vi "AutoCAD cmds.vi"(6 "AutoCAD cmd":T4, 8 "error in (no error)":errorcluster, 11 "UserInputs":T3) -> (0 "error out":errorcluster, 2 "IsQuiescent":bool)   [LabVIEW 2015, in "AguaClara Library.lvlib"]
uses:
  AguaClara Library.lvlib
  AutoCAD cmds.ctl
  user project design.ctl
  Variable cluster.ctl
  Design Request.ctl
panel:
  in  "Mathcad Output":T1
  out "DesignRequest out":T2
  in  "DesignRequest":T2
  out "new doc error":errorcluster
  out "Iterations":i32
  out "Visible":bool
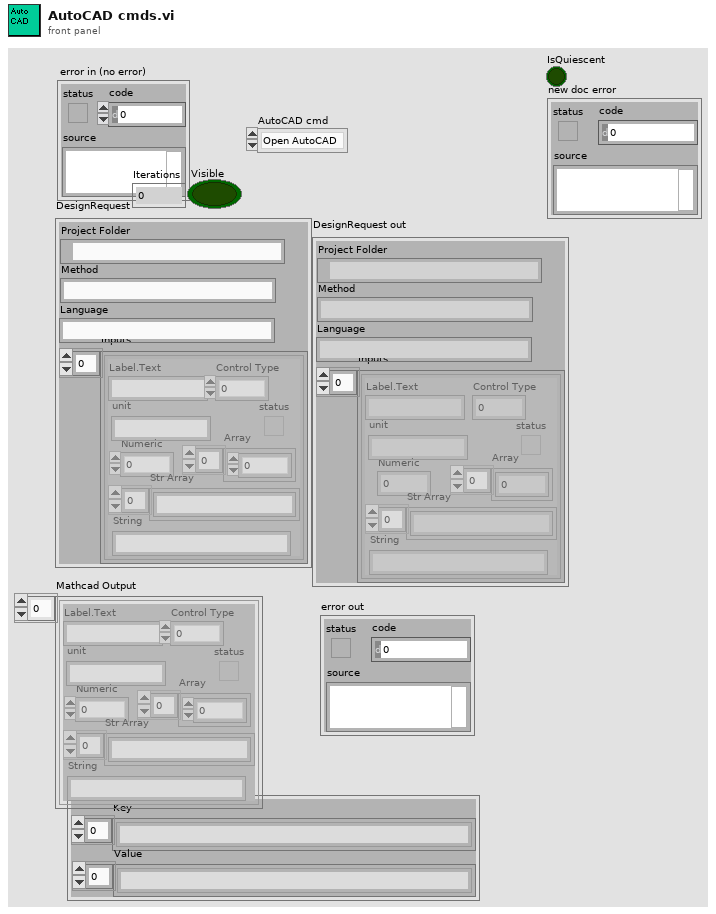
[diagram p1: front panel]
types:
  T1 = typedef "Variable cluster.ctl" = cluster{"Label.Text":string, "Control Type":u32, "Numeric":dbl, "Array":dbl[], "status":bool, "Str Array":string[], "String":string, "unit":string}[]
  T2 = typedef "Design Request.ctl" = cluster{"Project Folder":path, "Method":string, "Inputs":T1, "Language":string}
  T3 = typedef "user project design.ctl" = cluster{"Key":string[], "Value":string[]}
  T4 = typedef "AguaClara Library.lvlib/AutoCAD cmds.ctl" = enum16{"Open AutoCAD", "New Document", "Send Command", "Send Command Array", "Close Doc", "Quit"}
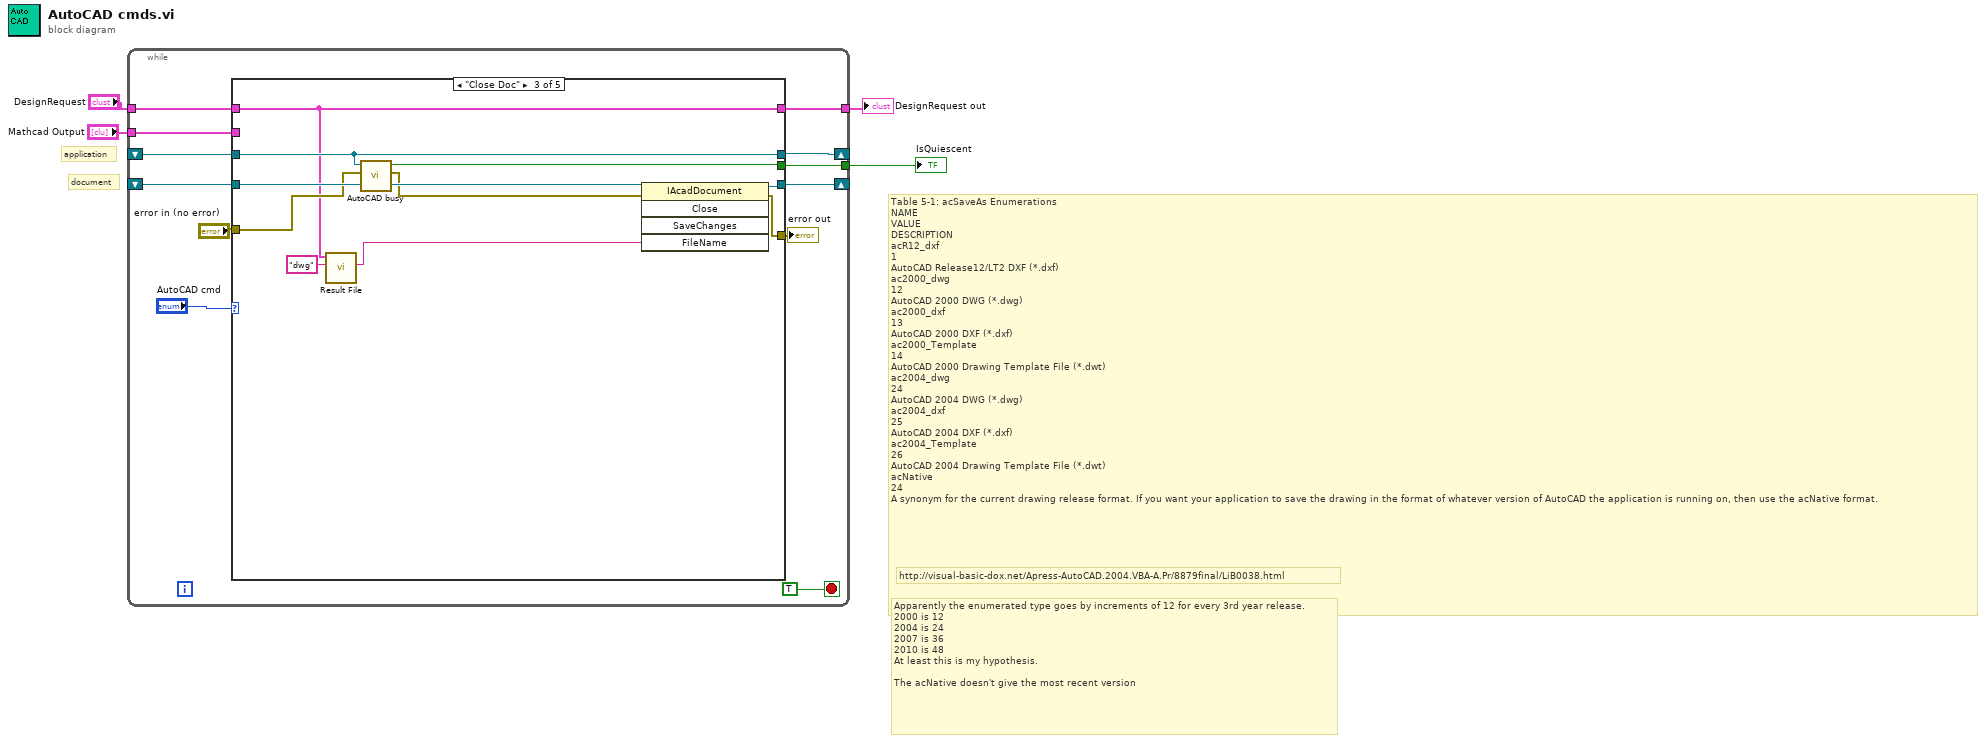
[diagram p0: block diagram]
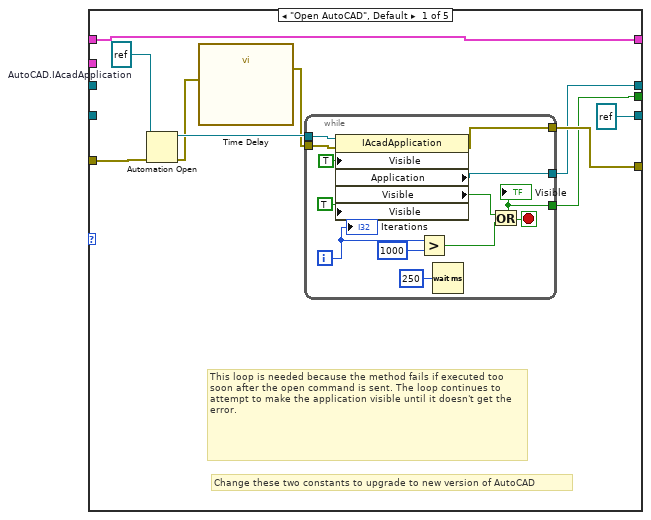
[diagram p2: hidden frame]
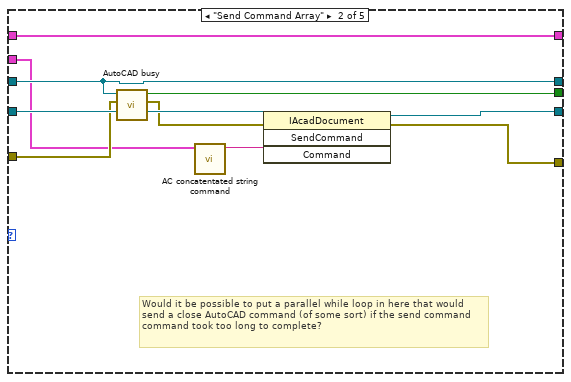
[diagram p3: hidden frame]
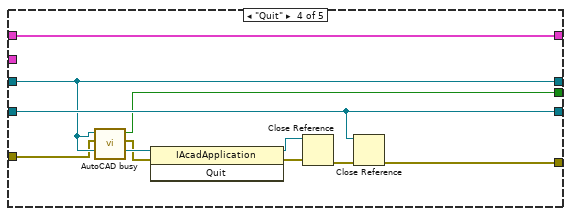
[diagram p4: hidden frame]
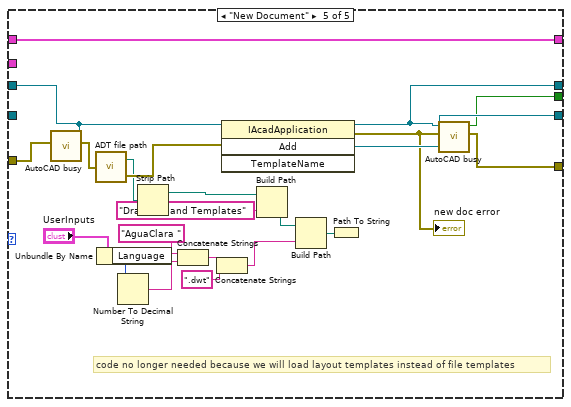
[diagram p5: hidden frame]
diagram:
  # "Apparently the enumerated type goes by increments of 12 for every 3rd year release.\n2000 is 12\n2004 is 24\n2007 is 36\n2010 is 48\nAt least this is my hypothesis. \n\nThe acNative doesn't give the most recent version"
  # "http://visual-basic-dox.net/Apress-AutoCAD.2004.VBA-A.Pr/8879final/LiB0038.html"
  # "Table 5-1: acSaveAs Enumerations\nNAME\nVALUE\nDESCRIPTION\nacR12_dxf\n1\nAutoCAD Release12/LT2 DXF (*.dxf)\nac2000_dwg\n12\nAutoCAD 2000 DWG (*.dwg)\nac2000_dxf\n13\nAutoCAD 2000 DXF (*.dxf)\nac2000_Template\n14\nAutoCAD 2000 Drawing Template File (*.dwt)\nac2004_dwg\n24\nAutoCAD 2004 DWG (*.dwg)\nac2004_dxf\n25\nAutoCAD 2004 DXF (*.dxf)\nac2004_Template\n26\nAutoCAD 2004 Drawing Template File (*.dwt)\nacNative\n24\nA synonym for the current drawing release format. If you want your application to save the drawing in the format of whatever version of AutoCAD the application is running on, then use the acNative format."
  # "document"
  # "application"
  n1 = while {
    shift-right: [w15] -> _
    shift-left: _ -> [w10]
    shift-right: [w12] -> _
    shift-left: _ -> [w11]
    tunnel: [w6] -> w4
    tunnel: "DesignRequest" -> [w7]
    tunnel: [w8] -> w2
    tunnel: "Mathcad Output" -> [w5]
    stop <- TRUE stop-if-true
    n2 = case shown="\"Close Doc\"" "AutoCAD cmd" {
      tunnel: [w21 w41 w55 w62 w87] -> w15
      tunnel: "error in (no error)" -> [w24 w45 w54 w61 w83]
      tunnel: [w22 w43 w56 w63 w86] -> w13
      tunnel: [refnum<k7> refnum ("AutoCAD.IAcadDocument") w47 w57 w64 w90] -> w12
      tunnel: w11 -> [_ w48 w58 w64 _]
      tunnel: w10 -> [_ w41 w55 w62 w88]
      tunnel: [w17 w39 w51 w68 w89] -> w8
      tunnel: w7 -> [w17 w39 w51 w68 w89]
      tunnel: [w20 w44 w52 w59 w85] -> w6
      tunnel: w5 -> [_ w40 _ _ _]
      frame "Open AutoCAD", Default {
        w25 = refnum<k7> refnum  # AutoCAD.IAcadApplication
        # "This loop is needed because the method fails if executed too soon after the open command is sent. The loop continues to attempt to make the application visible until it doesn't get the error."
        # "Change these two constants to upgrade to new version of AutoCAD"
        n3 = Automation Open(error in (no error)=w24, Automation Refnum=w25) -> (Automation Refnum=w23:refnum<k7>, error out=w19:errorcluster)  [unwired: 2 in]
        n4 = call "Time Delay"("error in (no error)"=w19) -> ("error out"=w18:errorcluster)  [unwired: 10 in]
        n5 = while {
          tunnel: w23 -> [w38]
          tunnel: w18 -> [w37]
          tunnel: [w32] -> w22
          tunnel: [w31] -> w21
          tunnel: [w28] -> w20
          i -> [w35]
          stop <- w36 stop-if-true
          n6 = property class="IAcadApplication"(reference=w38, error in=w37, "Visible"=TRUE, "Visible"=TRUE) -> (error out=w32:errorcluster, "Application"=w31:refnum<k7>, "Visible"=w28:bool)  [unwired: 1 out]
          "Visible" <- w28
          n7 = Greater?(x=w35, y=1000) -> (0:w33:bool)
          n8 = Wait (ms)(milliseconds to wait=u32 250) -> ()  [unwired: 1 out]
          n9 = Or(x=w28, y=w33) -> (x .or. y?=w36:bool)
          "Iterations" <- w35
        }
      }
      frame "Send Command Array" {
        # "Would it be possible to put a parallel while loop in here that would send a close AutoCAD command (of some sort) if the send command command took too long to complete?"
        n10 = call "AutoCAD busy.vi"("error in (no error)"=w45, "Application"=w41) -> ("error out"=w42:errorcluster, "IsQuiescent"=w44:bool)  [unwired: 4 in]
        n11 = call "AC concatentated string command.vi"("MathCAD results"=w40) -> ("AC concatenated string"=w46:string)  [unwired: 10 in]
        n12 = invoke class="IAcadDocument" method="SendCommand"(reference=w48, error in=w42, "Command"=w46) -> (reference out=w47:refnum<k7>, error out=w43:errorcluster)  [unwired: 1 in, 2 out]
      }
      frame "Close Doc" {
        n13 = call "Result File.vi"("File Type"="dwg", "DesignRequest"=w51) -> ("File string"=w49:string)  [unwired: 8 in, 1 out]
        n14 = call "AutoCAD busy.vi"("error in (no error)"=w54, "Application"=w55) -> ("error out"=w53:errorcluster, "IsQuiescent"=w52:bool)  [unwired: 4 in]
        n15 = invoke class="IAcadDocument" method="Close"(reference=w58, error in=w53, "FileName"=w49) -> (reference out=w57:refnum<k7>, error out=w56:errorcluster)  [unwired: 2 in, 3 out]
      }
      frame "Quit" {
        n16 = call "AutoCAD busy.vi"("error in (no error)"=w61, "Application"=w62) -> ("error out"=w60:errorcluster, "IsQuiescent"=w59:bool)  [unwired: 4 in]
        n17 = invoke class="IAcadApplication" method="Quit"(reference=w62, error in=w60) -> (reference out=w67:refnum<k7>, error out=w66:errorcluster)  [unwired: 1 in, 1 out]
        n18 = Close Reference(reference=w67, error in (no error)=w66) -> (error out=w65:errorcluster)
        n19 = Close Reference(reference=w64, error in (no error)=w65) -> (error out=w63:errorcluster)
      }
      frame "New Document" {
        # "code no longer needed because we will load layout templates instead of file templates"
        n20 = call "AutoCAD busy.vi"("error in (no error)"=w83, "Application"=w88) -> ("error out"=w82:errorcluster)  [unwired: 4 in, 1 out]
        n21 = call "ADT file path.vi"("error in"=w82) -> ("error out"=w81:errorcluster, "dup path"=w74:path)
        n22 = Unbundle By Name("UserInputs") -> ("Language"=w80:enum16{"English", "Español", "French"})
        n23 = Number To Decimal String(number=w80) -> (decimal integer string=w78:string)  [unwired: 1 in]
        n24 = Strip Path(path=w74) -> (stripped path=w73:path)  [unwired: 1 out]
        n25 = Concatenate Strings("AguaClara " ("section"), w78) -> (w77:string)
        n26 = Concatenate Strings(w77, ".dwt" ("string")) -> (w69:string)
        n27 = invoke class="IAcadApplication" method="Add"(reference=w88, error in=w81) -> (reference out=w87:refnum<k7>, error out=w84:errorcluster, "Add"=w90:refnum<k7>)  [unwired: 2 in, 1 out]
        "new doc error" <- w84
        n28 = Build Path(base path=w73, name or relative path="Drawings and Templates") -> (appended path=w71:path)
        n29 = Build Path(base path=w71, name or relative path=w69) -> (appended path=w70:path)
        n30 = Path To String(path=w70) -> ()  [unwired: 1 out]
        n31 = call "AutoCAD busy.vi"("error in (no error)"=w84, "Application"=w87) -> ("error out"=w86:errorcluster, "IsQuiescent"=w85:bool)  [unwired: 4 in]
      }
    }
    "error out" <- w13
  }
  "IsQuiescent" <- w4
  "DesignRequest out" <- w2
